vi "Read Tank Pressure and Temperatures.vi"(8 "error in (no error)":errorcluster, 9 "Pressure Units":T1=enum."PSIA", 10 "Temp Units":T1, 11 "Process Settings in":refnum<class "Process Settings.lvclass">) -> (0 "error out":errorcluster, 1 "Tank Pressure":dbl, 2 "Tank Temperature Cluster":T2, 3 "Process Settings out":refnum<class "Process Settings.lvclass">)   [LabVIEW 2017, in "Saturation.lvclass"]
uses:
  Saturation/Saturation.lvclass
  Process Settings/Process Settings.lvclass
  Saturation/Type Defs/Saturation Temps.ctl
  Process Settings/Type Defs/Units.ctl
  Hardware Settings/Type Defs/Hardware Types.ctl
  Process Settings/Process Settings.lvclass/Process Settings.ctl
  Process Settings/Accessors/Read Hardware Settings.vi
  Hardware Settings/Hardware Settings.lvclass
  Hardware Settings/Hardware Types/Generic/Generic Hardware.lvclass
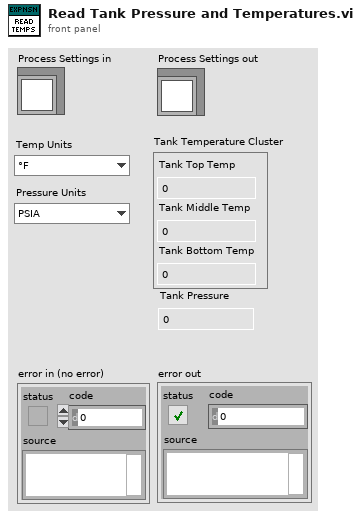
[diagram p1: front panel]
types:
  T1 = typedef "Process Settings.lvclass/Units.ctl" = enum16{"°F", "°C", "Seconds", "Minutes", "PSIA", "V"}
  T2 = typedef "Saturation.lvclass/Saturation Temps.ctl" = cluster{"Tank Top Temp":dbl, "Tank Middle Temp":dbl, "Tank Bottom Temp":dbl}
  T3 = typedef "Hardware Settings.lvclass/Hardware Types.ctl" = enum16{"Tank Chamber Pressure and Temperature", "Tank Valve Controls", "Motor On/Off and Direction Control", "Limit Switches", "IR Temperature", "Pneumatic Cylinder Actuation", "Expansion Temperature Setpoint"}
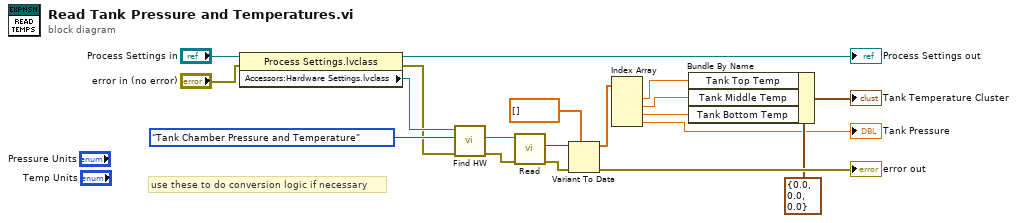
[diagram p0: block diagram]
diagram:
  # "use these to do conversion logic if necessary"
  n1 = property class="Process Settings.lvclass"(reference="Process Settings in", error in="error in (no error)") -> (reference out=→"Process Settings out":refnum<class "Process Settings.lvclass">, error out=w3:errorcluster, "Accessors:Hardware Settings.lvclass"=w6:refnum<class "Hardware Settings.lvclass">)
  n2 = call "Find HW.vi"("error in (no error)"=w3, "HW Item"=Hardware_Types."Tank Chamber Pressure and Temperature", "Hardware Settings in"=w6) -> ("error out"=w17:errorcluster, "Selected Hardware Out"=w14:refnum<class "Generic Hardware.lvclass">)  [unwired: 6 in, 1 out]
  n3 = call-dynamic "Read.vi"("error in (no error)"=w17, "Generic Hardware in"=w14) -> ("error out"=w18:errorcluster, "Output"=w15:variant)  [unwired: 7 in, 1 out]
  n4 = Variant To Data(error in=w18, type=dbl[] [], Variant=w15) -> (data=w16:dbl[], error out=→"error out":errorcluster)
  n5 = Index Array(array=w16) -> (element #1=w10:dbl, element #2=w9:dbl, element #3=w2:dbl, element #4=→"Tank Pressure":dbl)  [unwired: 4 in]
  n6 = Bundle By Name(cluster=T2 {"Tank Top Temp"=0.0, "Tank Middle Temp"=0.0, "Tank Bottom Temp"=0.0} ("System Cluster"), "Tank Top Temp"=w10, "Tank Middle Temp"=w9, "Tank Bottom Temp"=w2) -> (→"Tank Temperature Cluster":T2)
